vi "Add Meas Plugin Indicators - Multiple Converter.vi"(11 "error in":errorcluster) -> (15 "error out":errorcluster)   [LabVIEW 2021, in "Converter.lvlib"]
uses:
  Converter.lvlib
  Converter Reusables/Converter Reusables.lvlib
  Path Functions/Path Functions.lvlib
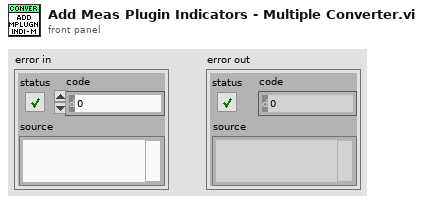
[diagram p1: front panel]
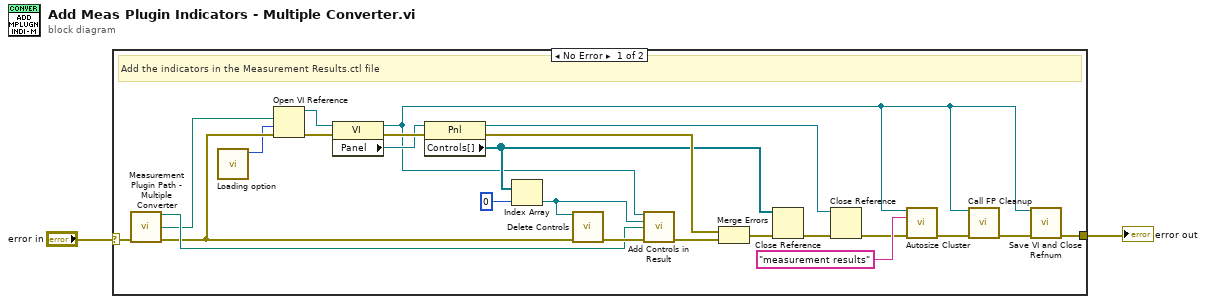
[diagram p0: block diagram]
diagram:
  n1 = case shown="No Error" "error in" {
    selector: "error in" -> [w7 w27]
    tunnel: [w5 w27] -> w2
    frame No Error {
      # "Add the indicators in the Measurement Results.ctl file"
      n2 = call "Measurement Plugin Path - Multiple Converter.vi"("error in"=w7) -> ("new code module"=w9:path, "result control"=w8:path, "error out"=w6:errorcluster)  [unwired: 2 in, 10 out]
      n3 = call "Loading option.vi"() -> ("options"=w4:i32)  [unwired: 11 in]
      n4 = Open VI Reference(vi path=w8, options=w4, error in (no error)=w6) -> (vi reference=w3:refnum<vi>, error out=w22:errorcluster)  [unwired: 3 in]
      n5 = property class="VI"(reference=w3, error in=w22) -> (reference out=w12:refnum<vi>, error out=w26:errorcluster, "Panel"=w23:refnum<vi>)
      n6 = property class="Pnl"(reference=w23, error in=w26) -> (reference out=w17:refnum<vi>, error out=w16:errorcluster, "Controls[]"=w15:refnum<vi>[])
      n7 = Index Array(array=w15, index=0) -> (element=w11:refnum<vi>)
      n8 = call "Delete Controls.vi"("control in"=w11, "error in"=w6) -> ("error out"=w10:errorcluster)  [unwired: 13 in]
      n9 = call "Add Controls in Result.vi"("vi reference"=w12, "result cluster"=w11, "new code module"=w9, "error in"=w10) -> ("error out"=w24:errorcluster)  [unwired: 11 in]
      n10 = Merge Errors(w16, w24) -> (w14:errorcluster)
      n11 = Close Reference(reference=w15, error in (no error)=w14) -> (error out=w13:errorcluster)
      n12 = Close Reference(reference=w17, error in (no error)=w13) -> (error out=w20:errorcluster)
      n13 = call "Autosize Cluster.vi"("vi refnum"=w12, "name"="measurement results" ("name/order"), "error in"=w20) -> ("error out"=w19:errorcluster)  [unwired: 12 in]
      n14 = call "Call FP Cleanup.vi"("vi"=w12, "error in"=w19) -> ("error out"=w18:errorcluster)  [unwired: 13 in]
      n15 = call "Save VI and Close Refnum.vi"("vi refnum"=w12, "error in"=w18) -> ("error out"=w5:errorcluster)  [unwired: 13 in]
    }
    frame Error {
    }
  }
  "error out" <- w2
